vi "Scale Problem Linear.vi"(8 "error in (no error)":errorcluster, 9 "Scaling limits":T3={"X lower"=-1.0, "X upper"=1.0, "Y lower"=nan, "Y upper"=nan}, 11 "Problem":T1) -> (0 "error out":errorcluster, 1 "ymaxmin":cluster{"ymax":dbl, "ymin":dbl}, 2 "xmaxmin":cluster{"min":dbl, "max":dbl}[](array[cluster]), 3 "Scaled problem":T1)   [LabVIEW 2014]
doc: "Scales the problem similarly to the svm-scale tool bundled with libsvm.\nAlways use the output from this VI to scale the test set instead of scaling individually."
uses:
  Libsvm Wrapper/Controls/svm_problem.ctl
  Libsvm Wrapper/Controls/svm_node.ctl
  Controls/Statemachine_ScaleProblem.ctl
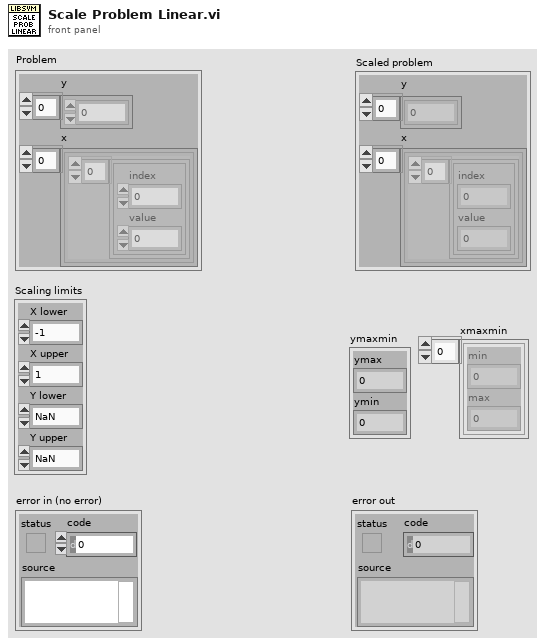
[diagram p1: front panel]
types:
  T1 = typedef "svm_problem.ctl" = cluster{"y":dbl[], "x":cluster{T2[]}[]}
  T2 = typedef "svm_node.ctl" = cluster{"index":i32, "value":dbl}
  T3 = cluster{"X lower":dbl, "X upper":dbl, "Y lower":dbl, "Y upper":dbl}
  T4 = typedef "Statemachine_ScaleProblem.ctl" = enum16{"Input verification: Limits", "Input verification: Ascending indices", "Find max/min index", "Find max/min features", "Scale", "Stop"}
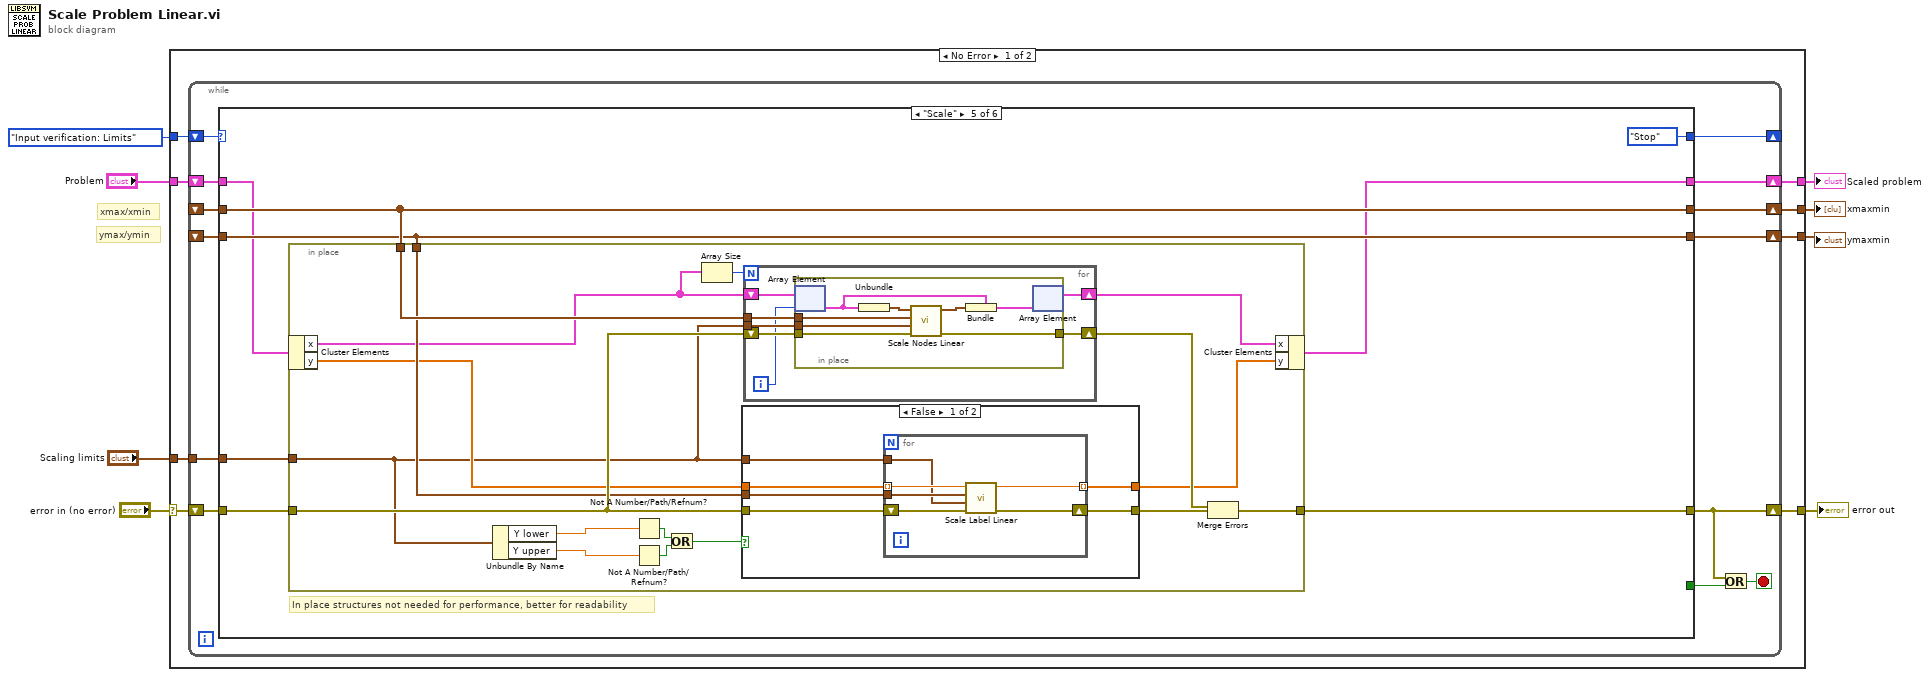
[diagram p0: block diagram]
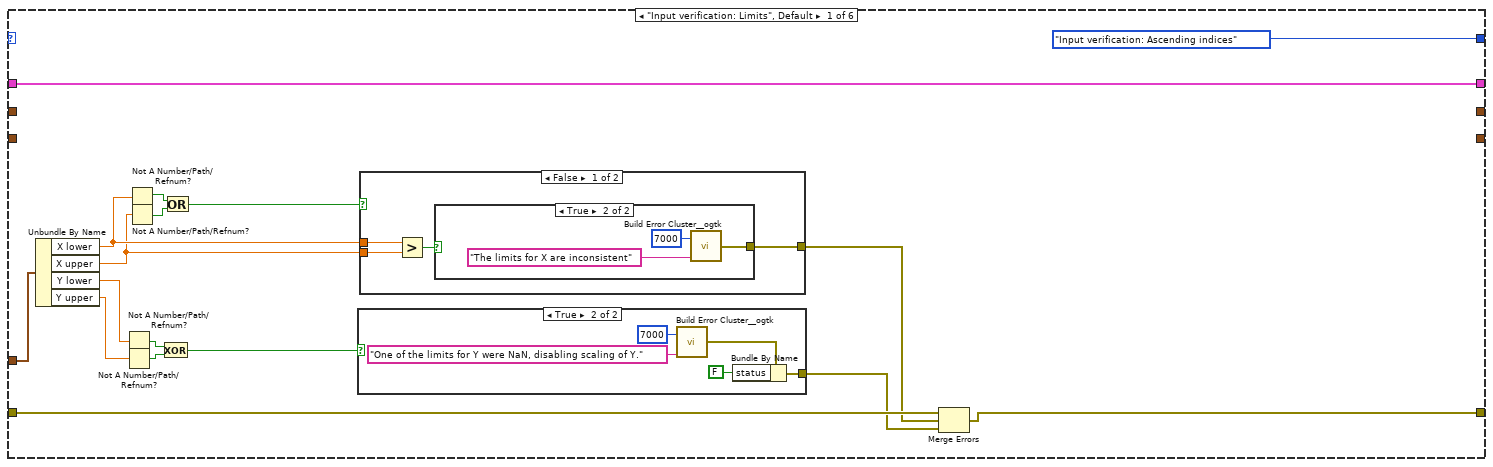
[diagram p2: hidden frame]
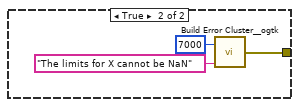
[diagram p5: hidden frame]
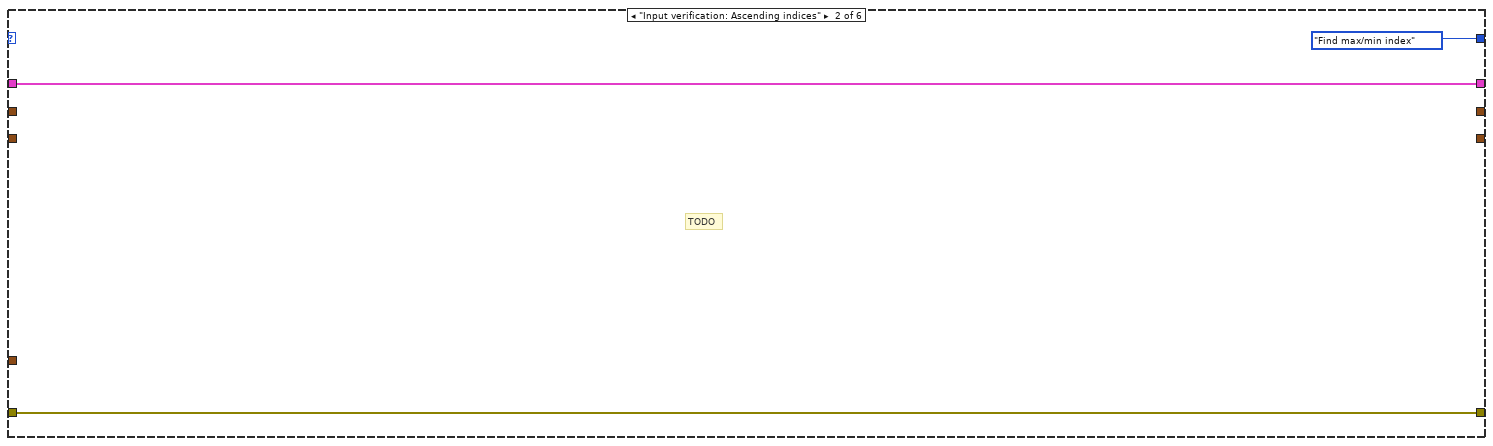
[diagram p6: hidden frame]
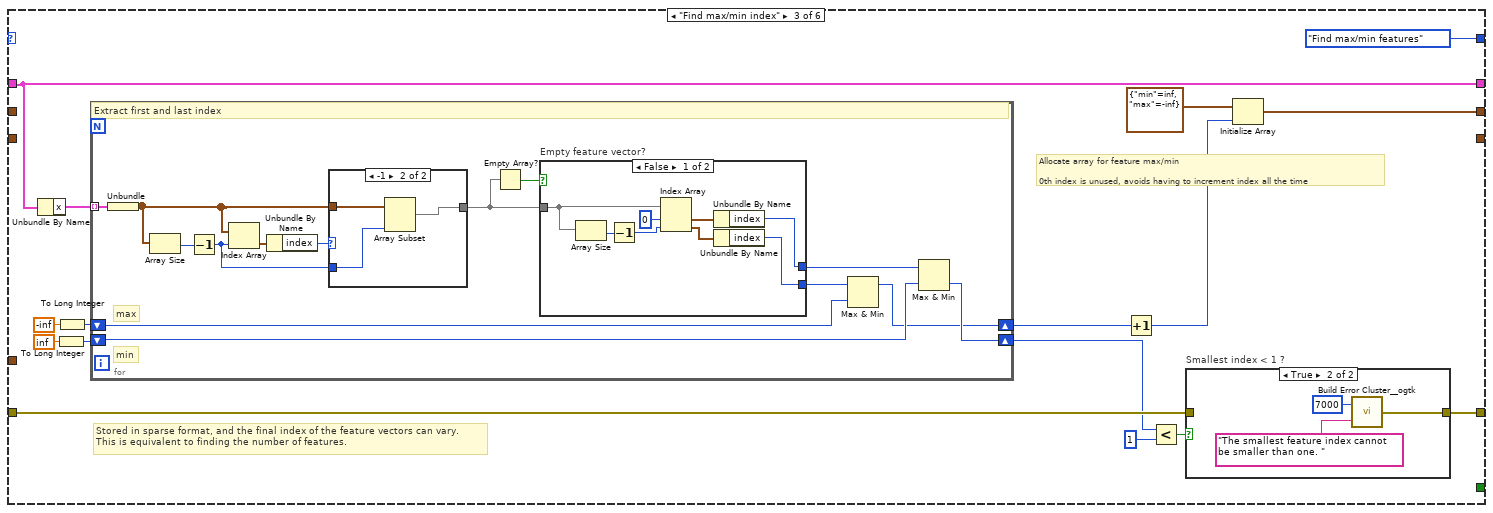
[diagram p7: hidden frame]
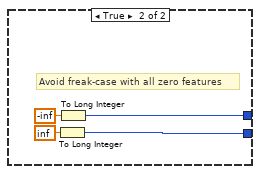
[diagram p10: hidden frame]
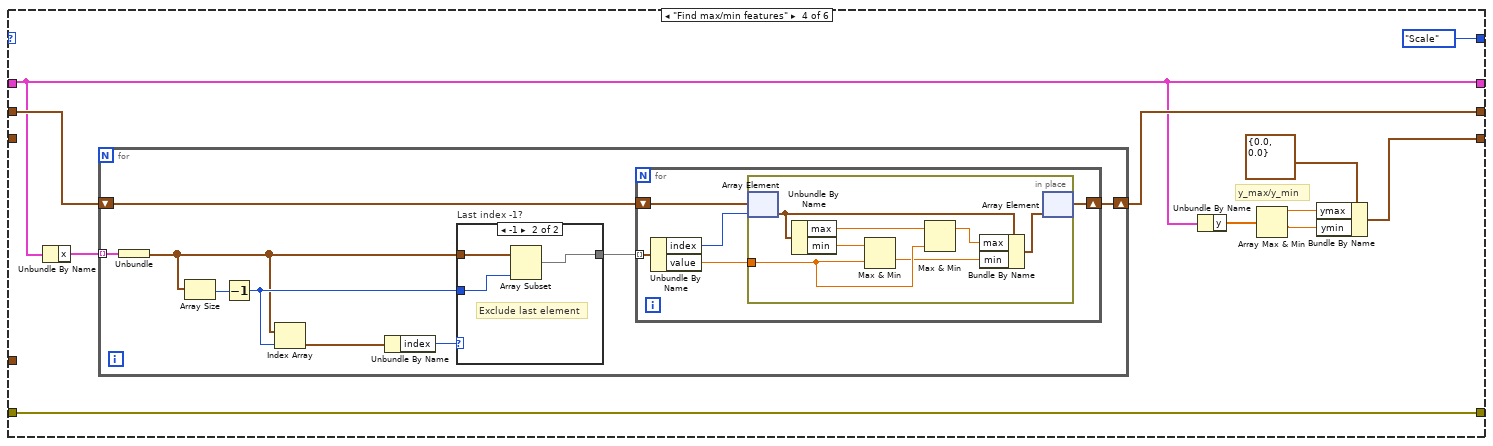
[diagram p11: hidden frame]
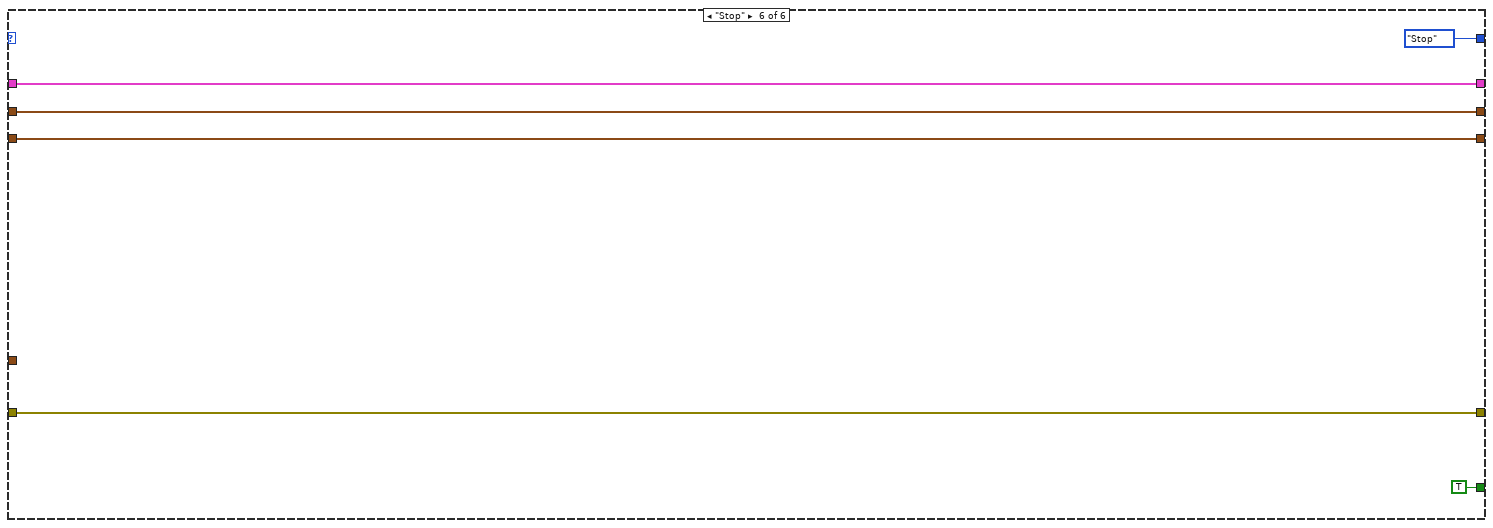
[diagram p14: hidden frame]
diagram:
  # "ymax/ymin"
  # "xmax/xmin"
  n1 = case shown="No Error" "error in (no error)" {
    selector: "error in (no error)" -> [w16 w211]
    tunnel: [w13 w211] -> w8
    tunnel: "Problem" -> [w9 _]
    tunnel: "Scaling limits" -> [w14 _]
    tunnel: Statemachine_ScaleProblem."Input verification: Limits" ("Statemachine_ScaleProblem") -> [w15 _]
    tunnel: [w12 _] -> w2
    tunnel: [w11 _] -> w3
    tunnel: [w10 _] -> w1
    frame No Error {
      n2 = while {
        shift-right: [w26] -> _
        shift-left: w15 -> [w29]
        tunnel: w14 -> [w28]
        shift-right: [w19] -> w13
        shift-left: w16 -> [w27]
        shift-right: [w25] -> w11
        shift-left: _ -> [w24]
        shift-right: [w23] -> w12
        shift-left: _ -> [w22]
        shift-right: [w21] -> w10
        shift-left: w9 -> [w20]
        stop <- w18 stop-if-true
        n3 = case shown="\"Scale\"" w29 {
          tunnel: w28 -> [w46 _ _ _ w157 _]
          tunnel: w27 -> [w35 w64 w72 w122 w156 w209]
          tunnel: [w32 w64 w73 w122 w155 w209] -> w19
          tunnel: [Statemachine_ScaleProblem."Input verification: Ascending indices" ("Statemachine_ScaleProblem") Statemachine_ScaleProblem."Find max/min index" ("Statemachine_ScaleProblem") Statemachine_ScaleProblem."Find max/min features" ("Statemachine_ScaleProblem") Statemachine_ScaleProblem."Scale" ("Statemachine_ScaleProblem") Statemachine_ScaleProblem."Stop" ("Statemachine_ScaleProblem") Statemachine_ScaleProblem."Stop" ("Statemachine_ScaleProblem")] -> w26
          tunnel: [_ _ w69 w123 w154 w208] -> w25
          tunnel: w24 -> [_ _ _ w124 w154 w208]
          tunnel: [_ _ _ w118 w153 w207] -> w23
          tunnel: w22 -> [_ _ _ _ w153 w207]
          tunnel: [w30 w62 w67 w116 w151 w206] -> w21
          tunnel: w20 -> [w30 w62 w67 w116 w152 w206]
          tunnel: [_ _ _ _ _ TRUE] -> w17
          frame "Input verification: Limits", Default {
            n4 = Unbundle By Name(w46) -> ("X lower"=w40:dbl, "X upper"=w39:dbl, "Y lower"=w44:dbl, "Y upper"=w45:dbl)
            n5 = Not A Number/Path/Refnum?(number/path/refnum=w44) -> (NaN/Path/Refnum?=w38:bool)
            n6 = Not A Number/Path/Refnum?(number/path/refnum=w45) -> (NaN/Path/Refnum?=w37:bool)
            n7 = Not A Number/Path/Refnum?(number/path/refnum=w40) -> (NaN/Path/Refnum?=w42:bool)
            n8 = Not A Number/Path/Refnum?(number/path/refnum=w39) -> (NaN/Path/Refnum?=w43:bool)
            n9 = Exclusive Or(1:w37, 2:w38) -> (0:w36:bool)
            n10 = Or(x=w42, y=w43) -> (x .or. y?=w41:bool)
            n11 = case shown="True" w36 {
              tunnel: [_ w47] -> w33
              frame False {
              }
              frame True {
                n12 = call <userlib>:"Build Error Cluster__ogtk.vi"("String to Prepend to source (\"\")"="One of the limits for Y were NaN, disabling scaling of Y." ("String to Prepend to source (\"\")"), "code"=7000) -> ("error out"=w49:errorcluster)
                n13 = Bundle By Name(cluster=w49, "status"=FALSE) -> (w47:errorcluster)
              }
            }
            n14 = case shown="False" w41 {
              tunnel: w40 -> [w54 _]
              tunnel: w39 -> [w53 _]
              tunnel: [w52 w59] -> w34
              frame False {
                n15 = Greater?(x=w54, y=w53) -> (0:w55:bool)
                n16 = case shown="True" w55 {
                  tunnel: [_ w56] -> w52
                  frame False {
                  }
                  frame True {
                    n17 = call <userlib>:"Build Error Cluster__ogtk.vi"("String to Prepend to source (\"\")"="The limits for X are inconsistent" ("String to Prepend to source (\"\")"), "code"=7000) -> ("error out"=w56:errorcluster)
                  }
                }
              }
              frame True {
                n18 = call <userlib>:"Build Error Cluster__ogtk.vi"("String to Prepend to source (\"\")"="The limits for X cannot be NaN" ("String to Prepend to source (\"\")"), "code"=7000) -> ("error out"=w59:errorcluster)
              }
            }
            n19 = Merge Errors(w35, w34, w33) -> (w32:errorcluster)
          }
          frame "Input verification: Ascending indices" {
            # "TODO"
          }
          frame "Find max/min index" {
            # "Allocate array for feature max/min\n\n0th index is unused, avoids having to increment index all the time"
            # "Stored in sparse format, and the final index of the feature vectors can vary.\nThis is equivalent to finding the number of features."
            n20 = Unbundle By Name(w67) -> ("x"=w80:cluster{T2[]}[])
            n21 = To Long Integer(number=inf) -> (32bit integer=w78:i32)
            n22 = To Long Integer(number=-inf) -> (32bit integer=w76:i32)
            n23 = for {
              tunnel: w80 -> [w98] mode=indexing
              shift-right: [w92] -> w66
              shift-left: w76 -> [w96]
              shift-right: [w93] -> w70
              shift-left: w78 -> [w94]
              # "min"
              # "max"
              # "Extract first and last index"
              n24 = Unbundle(w98) -> (w87:T2[])
              n25 = Array Size(array=w87) -> (size(s)=w90:i32)
              n26 = Decrement(x=w90) -> (x-1=w86:i32)
              n27 = Index Array(array=w87, index=w86) -> (element=w89:T2)
              n28 = Unbundle By Name(w89) -> ("index"=w88:i32)
              n29 = case shown="-1" w88 {
                tunnel: w87 -> [w99 w102]
                tunnel: w86 -> [_ w101]
                tunnel: [w99 w100] -> w85
                frame Default {
                }
                frame -1 {
                  n30 = Array Subset(array=w102, length=w101) -> (w100:T2[])  [unwired: 1 in]
                }
              }
              n31 = Empty Array?(array=w85) -> (empty?=w97:bool)
              n32 = case "Empty feature vector?" shown="False" w97 {
                tunnel: [w103 w111] -> w91
                tunnel: [w108 w112] -> w95
                tunnel: w85 -> [w106 _]
                frame False {
                  n33 = Array Size(array=w106) -> (size(s)=w105:i32)
                  n34 = Decrement(x=w105) -> (x-1=w104:i32)
                  n35 = Index Array(array=w106, index #1=0 ("index"), index #2=w104) -> (element #1=w109:T2, element #2=w107:T2)
                  n36 = Unbundle By Name(w109) -> ("index"=w108:i32)
                  n37 = Unbundle By Name(w107) -> ("index"=w103:i32)
                }
                frame True {
                  # "Avoid freak-case with all zero features"
                  n38 = To Long Integer(number=inf) -> (32bit integer=w111:i32)
                  n39 = To Long Integer(number=-inf) -> (32bit integer=w112:i32)
                }
              }
              n40 = Max & Min(x=w91, y=w96) -> (max(x,y)=w92:i32)  [unwired: 1 out]
              n41 = Max & Min(x=w95, y=w94) -> (min(x,y)=w93:i32)  [unwired: 1 out]
            }
            n42 = Increment(x=w66) -> (x+1=w65:i32)
            n43 = Less?(x=w70, y=1) -> (x < y?=w74:bool)
            n44 = case "Smallest index < 1 ?" shown="True" w74 {
              tunnel: [w81 w84] -> w73
              tunnel: w72 -> [w81 _]
              frame False {
              }
              frame True {
                n45 = call <userlib>:"Build Error Cluster__ogtk.vi"("String to Prepend to source (\"\")"="The smallest feature index cannot be smaller than one. " ("String to Prepend to source (\"\")"), "code"=7000) -> ("error out"=w84:errorcluster)
              }
            }
            n46 = Initialize Array(cluster{"min":dbl, "max":dbl} {"min"=inf, "max"=-inf}, w65) -> (w69:cluster{"min":dbl, "max":dbl}[])
          }
          frame "Find max/min features" {
            # "y_max/y_min"
            n47 = Unbundle By Name(w116) -> ("x"=w125:cluster{T2[]}[])
            n48 = for {
              tunnel: w125 -> [w134] mode=indexing
              shift-right: [w127] -> w123
              shift-left: w124 -> [w133]
              n49 = Unbundle(w134) -> (w126:T2[])
              n50 = Array Size(array=w126) -> (size(s)=w132:i32)
              n51 = Decrement(x=w132) -> (x-1=w129:i32)
              n52 = Index Array(array=w126, index=w129) -> (element=w131:T2)
              n53 = Unbundle By Name(w131) -> ("index"=w130:i32)
              n54 = case "Last index -1?" shown="-1" w130 {
                tunnel: w126 -> [w135 w138]
                tunnel: w129 -> [_ w137]
                tunnel: [w135 w136] -> w128
                frame Default {
                }
                frame -1 {
                  # "Exclude last element"
                  n55 = Array Subset(array=w138, length=w137) -> (w136:T2[])  [unwired: 1 in]
                }
              }
              n56 = for {
                tunnel: w128 -> [w143] mode=indexing
                shift-right: [w139] -> w127
                shift-left: w133 -> [w142]
                n57 = Unbundle By Name(w143) -> ("index"=w141:i32, "value"=w140:dbl)
                n58 = in-place {
                  in-place-border: w140 -> [w148]
                  n59 = in-place-array #1(w142, w141) -> (w147:cluster{"min":dbl, "max":dbl})
                  n60 = Unbundle By Name(w147) -> ("max"=w149:dbl, "min"=w150:dbl)
                  n61 = Max & Min(x=w150, y=w148) -> (min(x,y)=w145:dbl)  [unwired: 1 out]
                  n62 = Max & Min(x=w149, y=w148) -> (max(x,y)=w144:dbl)  [unwired: 1 out]
                  n63 = Bundle By Name(cluster=w147, "max"=w144, "min"=w145) -> (w146:cluster{"min":dbl, "max":dbl})
                  n64 = in-place-array #1(w146) -> (w139:cluster{"min":dbl, "max":dbl}[])  [unwired: 1 out]
                }
              }
            }
            n65 = Unbundle By Name(w116) -> ("y"=w115:dbl[])
            n66 = Array Max & Min(array=w115) -> (max value=w120:dbl, min value=w119:dbl)  [unwired: 2 out]
            n67 = Bundle By Name(cluster=cluster{"ymax":dbl, "ymin":dbl} {"ymax"=0.0, "ymin"=0.0}, "ymax"=w120, "ymin"=w119) -> (w118:cluster{"ymax":dbl, "ymin":dbl})
          }
          frame "Scale" {
            # "In place structures not needed for performance, better for readability"
            n68 = in-place {
              in-place-border: w157 -> [w159]
              in-place-border: w156 -> [w175]
              in-place-border: [w174] -> w155
              in-place-border: w154 -> [w166]
              in-place-border: w153 -> [w165]
              n69 = in-place-cluster #2(w152) -> ("x"=w161:cluster{T2[]}[], "y"=w164:dbl[])
              n70 = Unbundle By Name(w159) -> ("Y lower"=w171:dbl, "Y upper"=w170:dbl)
              n71 = Not A Number/Path/Refnum?(number/path/refnum=w171) -> (NaN/Path/Refnum?=w169:bool)
              n72 = Not A Number/Path/Refnum?(number/path/refnum=w170) -> (NaN/Path/Refnum?=w168:bool)
              n73 = Or(x=w169, y=w168) -> (x .or. y?=w167:bool)
              n74 = Array Size(array=w161) -> (size(s)=w162:i32)
              n75 = case shown="False" w167 {
                tunnel: w175 -> [w181 w188]
                tunnel: w164 -> [w180 w189]
                tunnel: w165 -> [w179 _]
                tunnel: [w178 w188] -> w173
                tunnel: [w177 w189] -> w163
                tunnel: w159 -> [w176 _]
                frame False {
                  n76 = for {
                    shift-right: [w186] -> w178
                    shift-left: w181 -> [w187]
                    tunnel: w180 -> [w185] mode=indexing
                    tunnel: w176 -> [w183]
                    tunnel: w179 -> [w184]
                    tunnel: [w182] -> w177 mode=indexing
                    n77 = call "Scale Label Linear.vi"("error in (no error)"=w187, "Scaling limits"=w183, "ymaxmin"=w184, "y"=w185) -> ("error out"=w186:errorcluster, "y scaled"=w182:dbl)  [unwired: 6 in]
                  }
                }
                frame True {
                  # "NaN y limit - do not perform scaling"
                }
              }
              n78 = for {
                N: w162 -> [_]
                tunnel: w166 -> [w195]
                shift-right: [w194] -> w172
                shift-left: w175 -> [w196]
                tunnel: w159 -> [w193]
                shift-right: [w190] -> w160
                shift-left: w161 -> [w192]
                i -> [w191]
                n79 = in-place {
                  in-place-border: w196 -> [w202]
                  in-place-border: w195 -> [w204]
                  in-place-border: [w201] -> w194
                  in-place-border: w193 -> [w203]
                  n80 = in-place-array #3(w192, w191) -> (w197:cluster{T2[]})
                  n81 = Unbundle(w197) -> (w200:T2[])
                  n82 = call "Scale Nodes Linear.vi"("error in (no error)"=w202, "Scaling limits"=w203, "xminmax"=w204, "x"=w200) -> ("error out"=w201:errorcluster, "x scaled"=w199:T2[])  [unwired: 6 in]
                  n83 = Bundle(cluster=w197, w199) -> (w198:cluster{T2[]})
                  n84 = in-place-array #3(w198) -> (w190:cluster{T2[]}[])  [unwired: 1 out]
                }
              }
              n85 = Merge Errors(w172, w173) -> (w174:errorcluster)
              n86 = in-place-cluster #2("x"=w160, "y"=w163) -> (w151:T1)
            }
          }
          frame "Stop" {
          }
        }
        n87 = Or(x=w19, y=w17) -> (x .or. y?=w18:bool)
      }
    }
    frame Error {
    }
  }
  "error out" <- w8
  "xmaxmin" <- w3
  "ymaxmin" <- w2
  "Scaled problem" <- w1
